vi "showCCD_dedicatedWindow.vi"(6 "ROI Descriptor":T1 {"Contours"."Type" items=["No Selection", "Point", "Line", "Rectangle", "Oval", "Polygon", "Freehand Region", "Annulus", "Unused2", "Unused3", "Broken Line", "Freehand Line", "Rotated Rectangle"]}, 8 "# Sat. Pix.":dbl=-1.0, 9 "Max":dbl=-1.0, 10 "Mean":dbl=-1.0, 11 "Refnum in":T2) -> ()   [LabVIEW 2023]
uses:
  <vilib>/vision/Image Controls.llb/IMAQ Image.ctl
panel:
  in  "Events list (all)":i32[](array[ring]) items=["No  event", "Click event", "Draw event", "Move event", "Size event", "Scroll event", "Activate event", "Close event", "Double click event"]
  out "Coordinates":i32[](array[numeric])
  out "Tool":i32(ring) items=["Point", "Line", "Rectangle", "Oval", "Polygon", "Freehand Region", "Annulus", "Rotated Rectangle", "Zoom", "Pan", "Broken Line", "Freehand Line"]
  out "Event":i32(ring) items=["No  event", "Click event", "Draw event", "Move event", "Size event", "Scroll event", "Activate event", "Close event", "Double click event"]
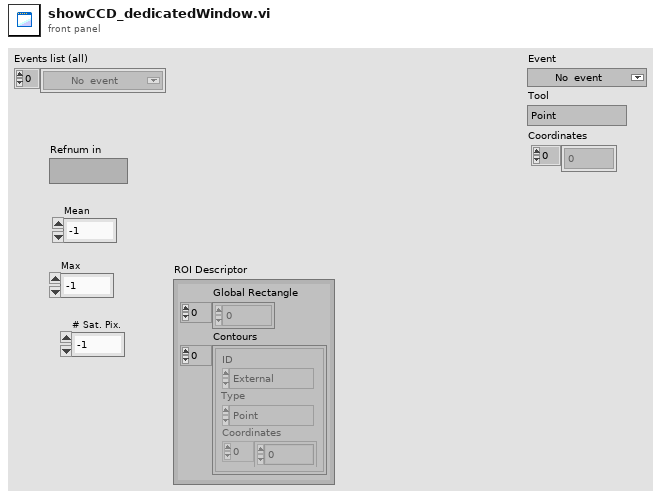
[diagram p1: front panel]
types:
  T1 = typedef "ROI Descriptor" = cluster{"Global Rectangle":i32[], "Contours":cluster{"ID":enum32{"External", "Internal"}, "Type":u32, "Coordinates":i32[]}[]}
  T2 = typedef "IMAQ Image.ctl" = refnum<image>
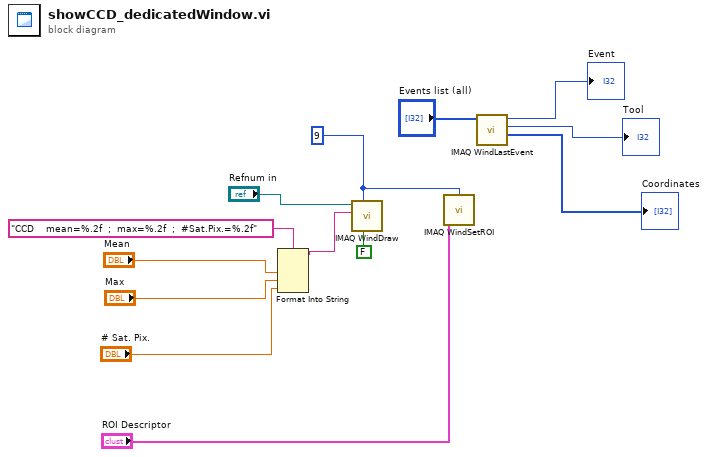
[diagram p0: block diagram]
diagram:
  w6 = 9 ("Window Number (0...15)")
  n1 = Format Into String(format string="CCD    mean=%.2f  ;  max=%.2f  ;  #Sat.Pix.=%.2f", "Mean", "Max", "# Sat. Pix.") -> (resulting string=w10:string)  [unwired: 2 in, 1 out]
  n2 = call "IMAQ WindDraw"("Resize to Image Size? (Y)"=FALSE, "Window Number (0...15)"=w6, "Title"=w10, "Image"="Refnum in") -> ()  [unwired: 6 in, 2 out]
  n3 = call "IMAQ WindSetROI"("Window Number (0...15)"=w6, "ROI Descriptor"="ROI Descriptor") -> ()  [unwired: 4 in, 1 out]
  n4 = call "IMAQ WindLastEvent"("Events list (all)"="Events list (all)") -> ("Coordinates"=→"Coordinates":i32[], "Tool"=→"Tool":i32, "Event"=→"Event":i32)  [unwired: 5 in, 3 out]
